vi "Get Results.vi"(8 "error in (no error)":errorcluster, 10 "Input Operations":T1(array[cluster]), 11 "Array":refnum<class "SimpleArithmetic.lvclass">[](array[class])) -> (0 "error out":errorcluster, 2 "Output Operations":T1(array[cluster]), 3 "Array Out":refnum<class "SimpleArithmetic.lvclass">[](array[class]))   [LabVIEW 2011]
uses:
  ClassDefinitions/SimpleClassWithMethods/SimpleArithmetic.lvclass
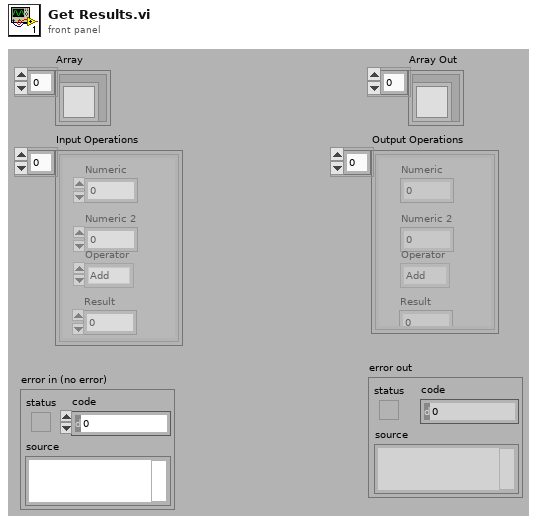
[diagram p1: front panel]
types:
  T1 = cluster{"Numeric":dbl, "Numeric 2":dbl, "Operator":enum16{"Add", "Divide", "Multiple", "Subtract"}, "Result":dbl}[]
  T2 = cluster{"Numeric":dbl, "Numeric 2":dbl, "Operator":enum16{"Add", "Divide", "Multiple", "Subtract"}, "Result":dbl}
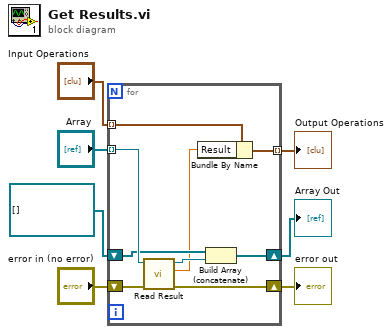
[diagram p0: block diagram]
diagram:
  n1 = for {
    tunnel: "Array" -> [w16] mode=indexing
    tunnel: "Input Operations" -> [w10] mode=indexing
    shift-right: [w11] -> w2
    shift-left: refnum<class "SimpleArithmetic.lvclass">[] [] ("Array") -> [w14]
    shift-right: [w12] -> w3
    shift-left: "error in (no error)" -> [w15]
    tunnel: [w8] -> w1 mode=indexing
    n2 = call "Read Result.vi"("error in (no error)"=w15, "SimpleArithmetic in"=w16) -> ("error out"=w12:errorcluster, "Result"=w9:dbl, "SimpleArithmetic out"=w13:refnum<class "SimpleArithmetic.lvclass">)  [unwired: 7 in]
    n3 = Bundle By Name(cluster=w10, "Result"=w9) -> (w8:T2)
    n4 = Build Array (concatenate)(w14, w13) -> (w11:refnum<class "SimpleArithmetic.lvclass">[])
  }
  "Array Out" <- w2
  "error out" <- w3
  "Output Operations" <- w1
